vi "YActor_Init.vi"(4 "ConstructorRef":refnum<vi>, 6 "ActorRef(EmptyRef=StandardActor)":refnum<vi>, 8 "ErrorIn":errorcluster, 11 "YActorIn":refnum<class "YActor.lvclass">) -> (0 "ErrorOut":errorcluster, 3 "YActorOut":refnum<class "YActor.lvclass">)   [LabVIEW 2021, in "YActor.lvclass"]
uses:
  YActor.lvclass
  YActor.lvclass/YActor.ctl
  ExeCmd_sync.vi
  private/SendCommand.vi
  private/WaitForReply.vi
  private/CreateLocalVI.vi
  private/ExeuteInlineVI.vi
  private/GetRemoteVIRef.vi
  private/GetNameOfVI.vi
  QuickCast.vi
  ExeCmd_async.vi
  ActorLightRun.vi
  private/VINameProperty.vi
  private/MessageCounter.vi
  InlineReferencePool.vi
  private/ExecuteVI.vi
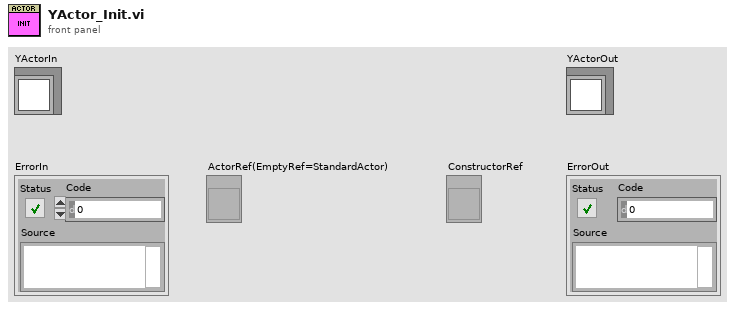
[diagram p1: front panel]
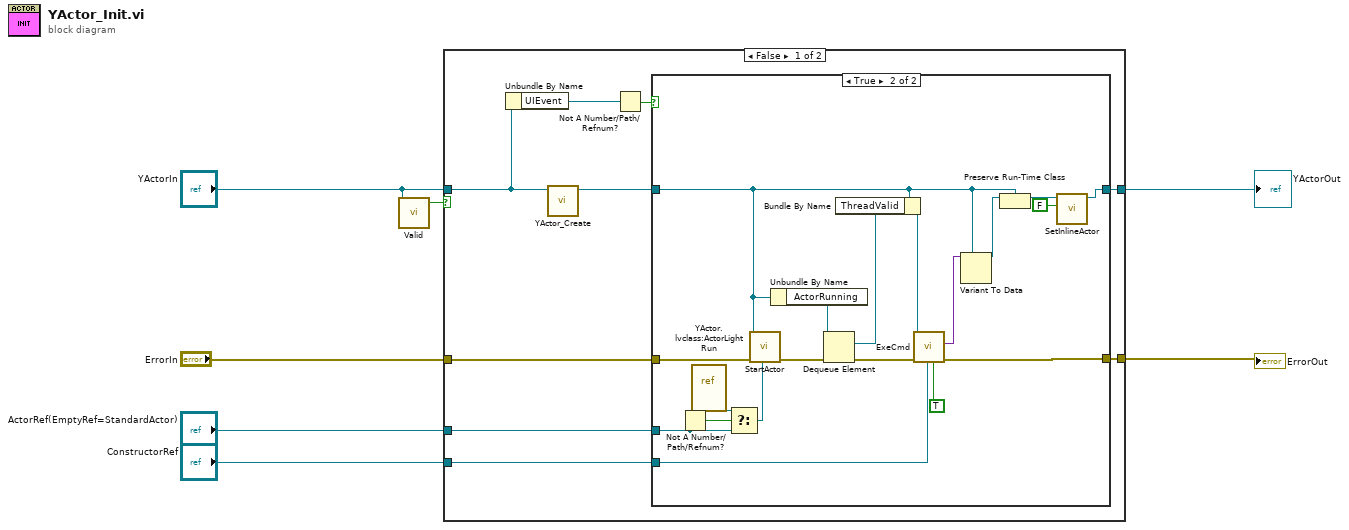
[diagram p0: block diagram]
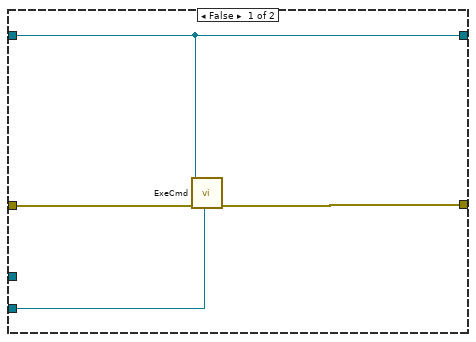
[diagram p2: hidden frame]
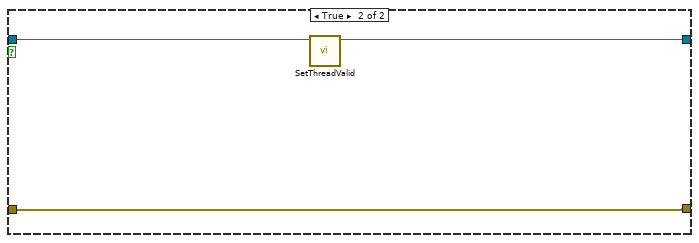
[diagram p3: hidden frame]
diagram:
  n1 = call "Valid.vi"("YActor in"="YActorIn") -> ("Valid"=w1:bool)  [unwired: 10 in]
  n2 = case shown="False" w1 {
    tunnel: "ConstructorRef" -> [w14 _]
    tunnel: "ActorRef(EmptyRef=StandardActor)" -> [w13 _]
    tunnel: "ErrorIn" -> [w16 w42]
    tunnel: [w15 w42] -> w6
    tunnel: "YActorIn" -> [w10 w40]
    tunnel: [w11 w41] -> w3
    frame False {
      n3 = Unbundle By Name(w10) -> ("UIEvent"=w8:refnum<user-event>)
      n4 = call "YActor_Create.vi"("YActorIn"=w10) -> ("YActorOut"=w12:refnum<class "YActor.lvclass">)  [unwired: 9 in, 1 out]
      n5 = Not A Number/Path/Refnum?(number/path/refnum=w8) -> (NaN/Path/Refnum?=w9:bool)
      n6 = case shown="True" w9 {
        tunnel: w14 -> [w18 w35]
        tunnel: w13 -> [_ w34]
        tunnel: w16 -> [w19 w39]
        tunnel: [w20 w38] -> w15
        tunnel: w12 -> [w17 w21]
        tunnel: [w17 w26] -> w11
        frame False {
          n7 = call-poly "ExeCmd.vi"("CmdVIRef"=w18, "ErrorIn"=w19, "YActorIn"=w17) -> ("ErrorOut"=w20:errorcluster)  [unwired: 8 in]
        }
        frame True {
          n8 = Not A Number/Path/Refnum?(number/path/refnum=w34) -> (NaN/Path/Refnum?=w33:bool)
          n9 = vi-ref "YActor.lvclass:ActorLightRun.vi"() -> (w32:refnum<vi>)
          n10 = Select(t=w32, s=w33, f=w34) -> (s? t:f=w31:refnum<vi>)
          n11 = call "StartActor.vi"("Reference"=w31, "ErrorIn"=w39, "YActorIn"=w21) -> ("ErrorOut"=w37:errorcluster)  [unwired: 8 in]
          n12 = Unbundle By Name(w21) -> ("ActorRunning"=w30:refnum<queue>)
          n13 = Dequeue Element(queue=w30, error in (no error)=w37) -> (element=w28:refnum<queue>, error out=w36:errorcluster)  [unwired: 1 in, 2 out]
          n14 = Bundle By Name(cluster=w21, "ThreadValid"=w28) -> (w29:refnum<class "YActor.lvclass">)
          n15 = call-poly "ExeCmd.vi"("HighPrio"=TRUE ("High Prio"), "CmdVIRef"=w35, "ErrorIn"=w36, "YActorIn"=w29) -> ("ErrorOut"=w38:errorcluster, "ReplyData"=w24:variant)  [unwired: 5 in, 1 out]
          n16 = Variant To Data(type=w21, Variant=w24) -> (data=w23:refnum<class "YActor.lvclass">)  [unwired: 1 in, 1 out]
          n17 = Preserve Run-Time Class(object in=w23, 2:w21) -> (object out=w22:refnum<class "YActor.lvclass">)  [unwired: 1 in, 1 out]
          n18 = call "SetInlineActor.vi"("Inline (T)"=FALSE, "YActor in"=w22) -> ("YActor out"=w26:refnum<class "YActor.lvclass">)  [unwired: 8 in, 1 out]
        }
      }
    }
    frame True {
      n19 = call "SetThreadValid.vi"("YActor in"=w40) -> ("YActor out"=w41:refnum<class "YActor.lvclass">)  [unwired: 10 in]
    }
  }
  "YActorOut" <- w3
  "ErrorOut" <- w6
